vi "IPS-Stop.vi"(2 "error in (no error)":errorcluster, 3 "Stop":bool) -> (0 "error out":errorcluster, 1 "Antwort":string)   [LabVIEW 2009]
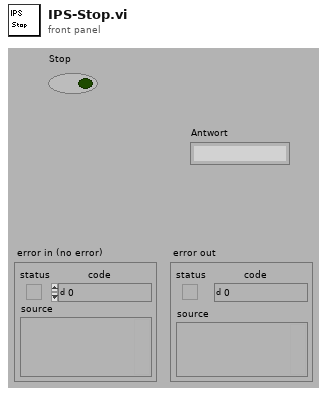
[diagram p1: front panel]
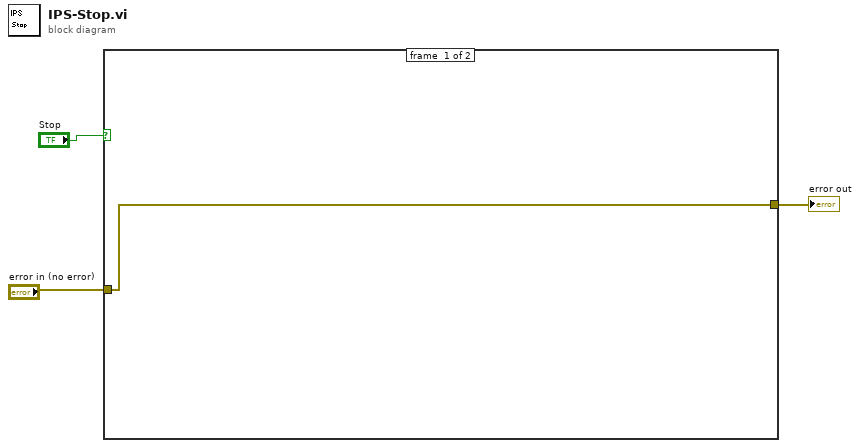
[diagram p0: block diagram]
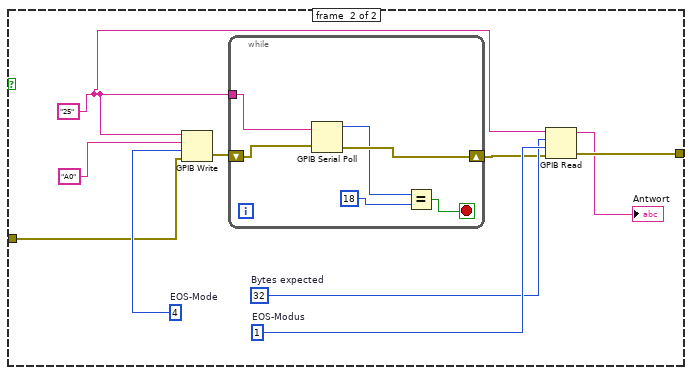
[diagram p2: hidden frame]
diagram:
  n1 = case shown="True" "Stop" {
    tunnel: "error in (no error)" -> [w4 w7]
    tunnel: [w4 w6] -> w1
    frame #0 {
    }
    frame #1 {
      w8 = "25"
      w14 = 1  # EOS-Modus
      w13 = 32  # Bytes expected
      w12 = 4  # EOS-Mode
      n2 = GPIB Write(0:w8, 1:"A0", 2:w12, 3:w7) -> (6:w11:errorcluster)  [unwired: 1 in, 1 out]
      n3 = while {
        shift-right: [w19] -> w10
        shift-left: w11 -> [w20]
        tunnel: w8 -> [w18]
        stop <- w17 stop-if-true
        n4 = GPIB Serial Poll(0:w18, 1:w20) -> (2:w15:i16, 4:w19:errorcluster)  [unwired: 1 out]
        n5 = Equal?(x=w15, y=18) -> (x = y?=w17:bool)
      }
      n6 = GPIB Read(0:w8, 1:w13, 2:w14, 3:w10) -> (5:→"Antwort":string, 7:w6:errorcluster)  [unwired: 1 in, 1 out]
    }
  }
  "error out" <- w1
